vi "生成CODMn data (子VI).vi"() -> (3 "data":T1)   [LabVIEW 2016, in "斯坦道CODMn.lvlib"]
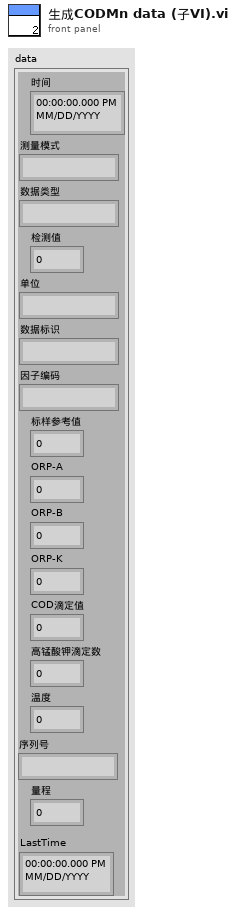
[diagram p1: front panel]
types:
  T1 = cluster{"时间":timestamp, "测量模式":string, "数据类型":string, "检测值":sgl, "单位":string, "数据标识":string, "因子编码":string, "标样参考值":sgl, "ORP-A":sgl, "ORP-B":sgl, "ORP-K":sgl, "COD滴定值":sgl, "高锰酸钾滴定数":sgl, "温度":sgl, "序列号":string, "量程":sgl, "LastTime":timestamp}
  T2 = cluster{"运行模式":enum16{"维护模式", "常规模式", "应急模式", "质控模式"}}
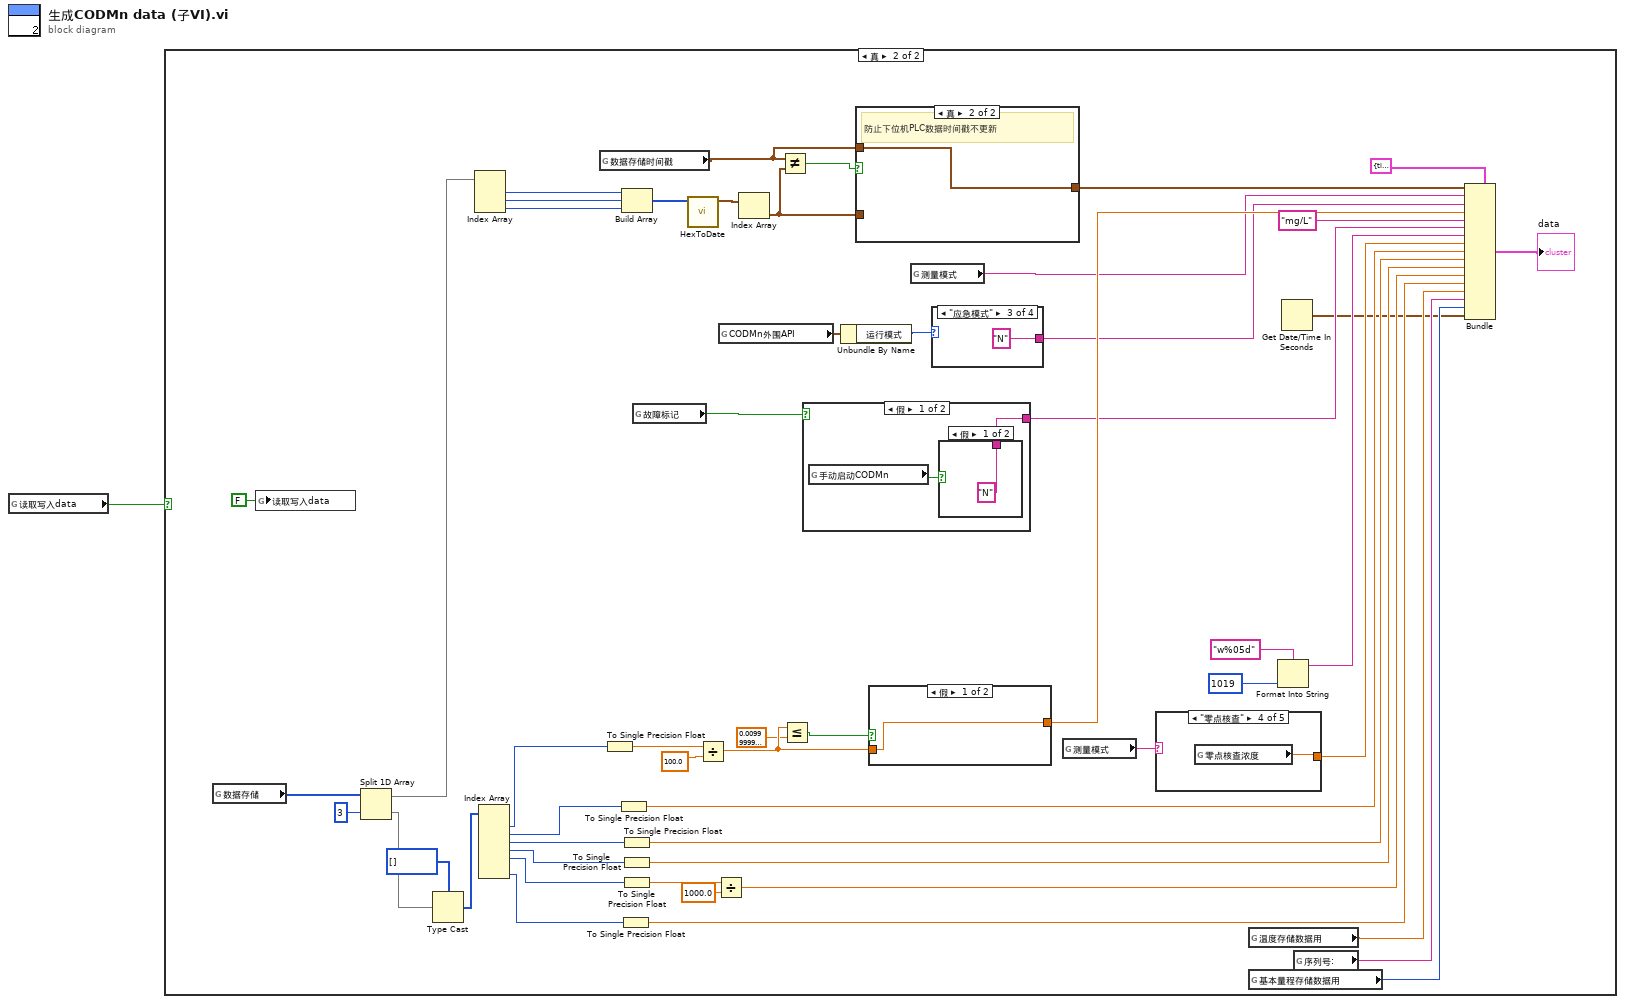
[diagram p0: block diagram]
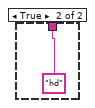
[diagram p4: hidden frame]
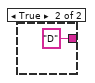
[diagram p5: hidden frame]
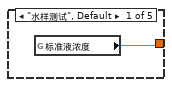
[diagram p6: hidden frame]
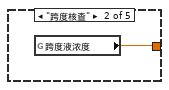
[diagram p7: hidden frame]
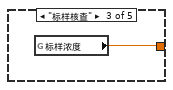
[diagram p8: hidden frame]
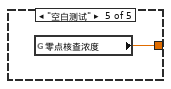
[diagram p9: hidden frame]
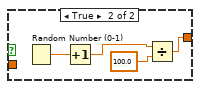
[diagram p10: hidden frame]
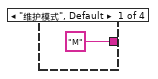
[diagram p11: hidden frame]
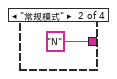
[diagram p12: hidden frame]
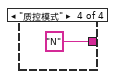
[diagram p13: hidden frame]
diagram:
  n1 = global read "COD读取DATA全局.vi" "读取写入data"() -> (w1:bool)
  n2 = case shown="真" w1 {
    frame False {
    }
    frame True {
      n3 = global read "COD读取DATA全局.vi" "数据存储"() -> (w9:u16[])
      n4 = global write "COD读取DATA全局.vi" "读取写入data"(FALSE ("读取写入data")) -> ()
      n5 = Split 1D Array(array=w9, index=3 ("索引")) -> (first subarray=w13:u16[], second subarray=w8:u16[])
      n6 = Type Cast(type=i16[] [], x=w8) -> (*(type *) &x=w7:i16[])
      n7 = Index Array(array=w13) -> (element #1=w15:u16, element #2=w16:u16, element #3=w17:u16)  [unwired: 3 in]
      n8 = Index Array(array=w7) -> (element #1=w41:i16, element #2=w19:i16, element #3=w20:i16, element #4=w21:i16, element #5=w22:i16, element #7=w51:i16)  [unwired: 7 in, 1 out]
      n9 = global read "COD读取DATA全局.vi" "数据存储时间戳"() -> (w52:timestamp)
      n10 = To Single Precision Float(number=w41) -> (single precision float=w39:sgl)
      n11 = To Single Precision Float(number=w19) -> (single precision float=w31:sgl)
      n12 = To Single Precision Float(number=w51) -> (single precision float=w36:sgl)
      n13 = Build Array(w15, w16, w17) -> (w18:u16[])
      n14 = To Single Precision Float(number=w20) -> (single precision float=w30:sgl)
      n15 = To Single Precision Float(number=w21) -> (single precision float=w29:sgl)
      n16 = To Single Precision Float(number=w22) -> (single precision float=w25:sgl)
      n17 = global read "COD读取DATA全局.vi" "故障标记"() -> (w54:bool)
      n18 = call "HexToDate.vi"("数组"=w18) -> ("DATE"=w14:timestamp[])  [unwired: 10 in]
      n19 = Divide(x=w39, y=sgl 100.0) -> (x/y=w40:sgl)
      n20 = Divide(x=w25, y=sgl 1000.0) -> (x/y=w28:sgl)
      n21 = global read "CODMN外部API.vi" "CODMn外围API"() -> (w44:T2)
      n22 = Index Array(array=w14) -> (element=w47:timestamp)  [unwired: 1 in]
      n23 = Not Equal?(x=w52, y=w47) -> (x != y?=w48:bool)
      n24 = Less Or Equal?(x=w40, y=sgl 0.01) -> (x <= y?=w38:bool)
      n25 = case shown="假" w54 {
        tunnel: [w58 "D" ("数据标识")] -> w33
        frame False {
          n26 = global read "CODMN外部API.vi" "手动启动CODMn"() -> (w57:bool)
          n27 = case shown="假" w57 {
            tunnel: ["N" ("数据标识") "hd" ("数据标识")] -> w58
            frame False {
            }
            frame True {
            }
          }
        }
        frame True {
        }
      }
      n28 = Unbundle By Name(w44) -> ("运行模式"=w45:enum16{"维护模式", "常规模式", "应急模式", "质控模式"})
      n29 = case "条件结构" shown="真" w48 {
        tunnel: w47 -> [w55 _]
        tunnel: w52 -> [_ w56]
        tunnel: [w55 w56] -> w49
        frame False {
        }
        frame True {
          # "防止下位机PLC数据时间戳不更新"
        }
      }
      n30 = case shown="假" w38 {
        tunnel: [w67 w68] -> w50
        tunnel: w40 -> [w67 _]
        frame False {
        }
        frame True {
          n31 = Random Number (0-1)() -> (number: 0 to 1=w71:dbl)
          n32 = Increment(x=w71) -> (x+1=w69:dbl)
          n33 = Divide(x=w69, y=sgl 100.0) -> (x/y=w68:dbl)
        }
      }
      n34 = global read "COD测量模式全局.vi" "测量模式"() -> (w46:string)
      n35 = case shown="\"应急模式\"" w45 {
        tunnel: ["M" ("单位") "N" ("单位") "N" ("单位") "N" ("单位")] -> w35
        frame "维护模式", Default {
        }
        frame "常规模式" {
        }
        frame "应急模式" {
        }
        frame "质控模式" {
        }
      }
      n36 = global read "COD测量模式全局.vi" "测量模式"() -> (w42:string)
      n37 = case shown="\"零点核查\"" w42 {
        tunnel: [w62 w63 w64 w65 w66] -> w43
        frame "水样测试", Default {
          n38 = global read "COD浓度全局变量.vi" "标准液浓度"() -> (w62:dbl)
        }
        frame "跨度核查" {
          n39 = global read "CODMn断电保存全局变量.vi" "跨度液浓度"() -> (w63:dbl)
        }
        frame "标样核查" {
          n40 = global read "CODMn断电保存全局变量.vi" "标样浓度"() -> (w64:dbl)
        }
        frame "零点核查" {
          n41 = global read "CODMn断电保存全局变量.vi" "零点核查浓度"() -> (w65:dbl)
        }
        frame "空白测试" {
          n42 = global read "CODMn断电保存全局变量.vi" "零点核查浓度"() -> (w66:dbl)
        }
      }
      n43 = global read "COD读取DATA全局.vi" "温度存储数据用"() -> (w53:dbl)
      n44 = global read "COD读取DATA全局.vi" "基本量程存储数据用"() -> (w3:enum16{"L", "H"})
      n45 = Format Into String(format string="w%05d" ("格式字符串"), u32 1019 ("因子编码")) -> (resulting string=w32:string)  [unwired: 2 in, 1 out]
      n46 = Get Date/Time In Seconds() -> (seconds since 1Jan1904=w2:timestamp)
      n47 = global read "COD读取DATA全局.vi" "序列号:"() -> (w4:string)
      n48 = Bundle(cluster=T1 {"时间"=timestamp(0 s since 1904-01-01), "测量模式"="", "数据类型"="", "检测值"=0.0, "单位"="", "数据标识"="", "因子编码"="", "标样参考值"=0.0, "ORP-A"=0.0, "ORP-B"=0.0, "ORP-K"=0.0, "COD滴定值"=0.0, "高锰酸钾滴定数"=0.0, "温度"=0.0, "序列号"="", "量程"=0.0, "LastTime"=timestamp(0 s since 1904-01-01)} ("data"), "时间"=w49, "测量模式"=w46, "数据类型"=w35, "检测值"=w50, "单位"="mg/L", "数据标识"=w33, "因子编码"=w32, "标样参考值"=w43, "ORP-A"=w31, "ORP-B"=w30, "ORP-K"=w29, "COD滴定值"=w28, "高锰酸钾滴定数"=w36, "温度"=w53, "序列号"=w4, "量程"=w3, "LastTime"=w2) -> (→"data":T1)
    }
  }
